vi "PDL_Process_AndSave.vi"(6 "Mergedata_struct":refnum<k24>[](array[refnum]), 7 "PDLSTS":refnum<k24>, 8 "错误输入（无错误）":errorcluster, 10 "PCU":refnum<k24>, 11 "chksavemu":bool) -> (0 "错误输出":errorcluster)   [LabVIEW 2017]
doc: "Save Measurement data"
uses:
  D:/test/PDLSTS/LV_PDL_Sample/DLL/STSProcess.dll
  DLL/STSProcess.dll
  D:/test/PDLSTS/LV_PDL_Sample/DLL/InstrumentDLL.dll
  DLL/InstrumentDLL.dll
panel:
  in  "SOPIL":dbl[][](array[numeric])
  in  "get_struct":refnum<k24>
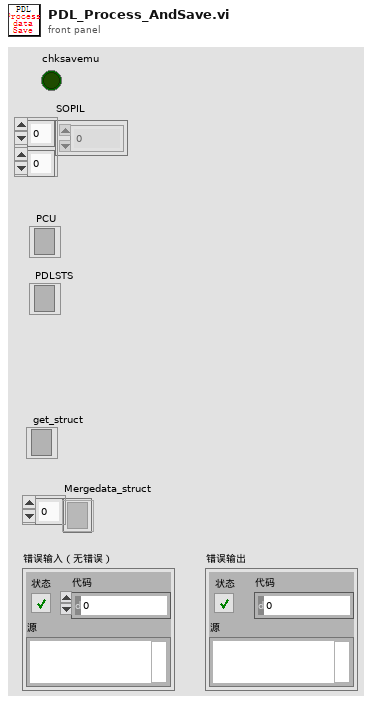
[diagram p1: front panel]
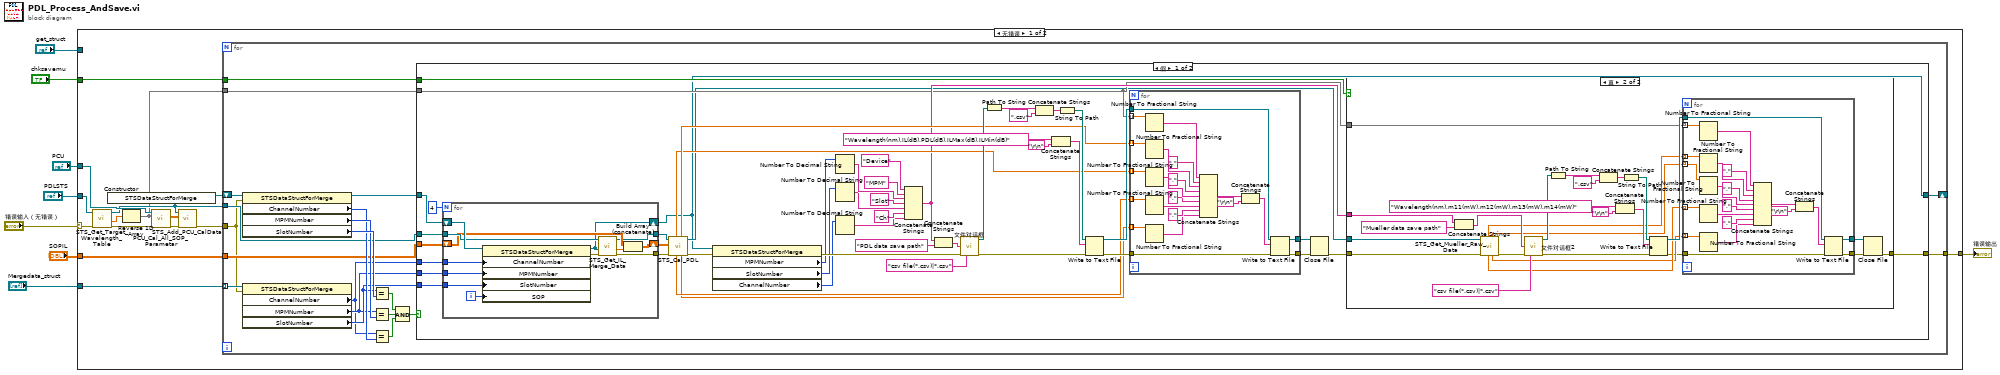
[diagram p0: block diagram]
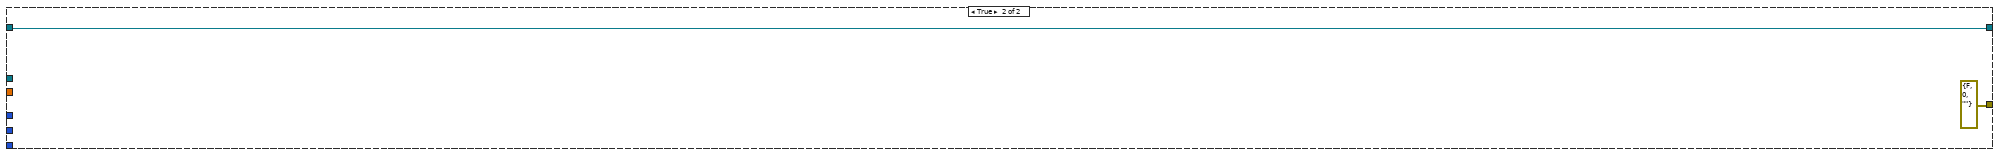
[diagram p3: hidden frame]
diagram:
  n1 = case shown="无错误" "错误输入（无错误）" {
    selector: "错误输入（无错误）" -> [w13 w177]
    tunnel: "Mergedata_struct" -> [w23 _]
    tunnel: "PDLSTS" -> [w22 _]
    tunnel: "PCU" -> [w20 _]
    tunnel: "get_struct" -> [_ _]
    tunnel: "SOPIL" -> [w16 _]
    tunnel: [w15 w177] -> w2
    tunnel: "chksavemu" -> [w12 _]
    frame No Error {
      n2 = call "STS_Get_Target_Wavelength_Table.vi"("错误输入（无错误）"=w13, ".NET引用句柄输入"=w22) -> ("error out"=w21:errorcluster, "wavelengths"=w10:dbl[], "引用输出"=w17:refnum<k24>)  [unwired: 7 in]
      n3 = constructor class="STSDataStructForMerge"() -> (reference out=w11:refnum<k24>)  [unwired: 3 in, 2 out]
      n4 = Reverse 1D Array(array=w10) -> (reversed array=w9:dbl[])
      n5 = call "PCU_Cal_All_SOP_Parametar.vi"("error in (no error)"=w21, "wave"=w9, ".NET Reference in"=w20) -> ("error out"=w19:errorcluster, "result out"=w18:sgl[][][])  [unwired: 6 in, 1 out]
      n6 = call "STS_Add_PCU_CalData.vi"("错误输入（无错误）"=w19, "errorArray"=w18, "STSProcess.PDLSTS"=w17) -> ("错误输出"=w14:errorcluster)  [unwired: 7 in, 1 out]
      n7 = for {
        tunnel: w17 -> [w31]
        tunnel: w23 -> [w43] mode=indexing
        tunnel: w16 -> [w30]
        tunnel: w9 -> [w29]
        tunnel: [w28] -> w15
        tunnel: w14 -> [w27]
        tunnel: w12 -> [w26]
        shift-right: [w25] -> _
        shift-left: w11 -> [w42]
        n8 = property class="STSDataStructForMerge"(reference=w42, error in=w27) -> (reference out=w24:refnum<k24>, "ChannelNumber"=w39:i32, "MPMNumber"=w40:i32, "SlotNumber"=w41:i32)  [unwired: 1 out]
        n9 = property class="STSDataStructForMerge"(reference=w43, error in=w27) -> ("ChannelNumber"=w32:i32, "MPMNumber"=w33:i32, "SlotNumber"=w34:i32)  [unwired: 2 out]
        n10 = Equal?(x=w34, y=w41) -> (x = y?=w38:bool)
        n11 = Equal?(x=w33, y=w40) -> (x = y?=w37:bool)
        n12 = Equal?(x=w32, y=w39) -> (x = y?=w36:bool)
        n13 = Compound Arithmetic op=AND ("复合运算")(w38, w37, w36) -> (w35:bool)
        n14 = case shown="假" w35 {
          tunnel: w24 -> [w91 w175]
          tunnel: w34 -> [w90 _]
          tunnel: w33 -> [w89 _]
          tunnel: w32 -> [w88 _]
          tunnel: w31 -> [w87 _]
          tunnel: w30 -> [w86 _]
          tunnel: w29 -> [w46 _]
          tunnel: [w48 errorcluster {"status"=FALSE, "code"=0, "source"=""} ("error out")] -> w28
          tunnel: w26 -> [w52 _]
          tunnel: [w44 w175] -> w25
          frame False {
            n15 = for {
              N: 4 -> [_]
              tunnel: w90 -> [w172]
              tunnel: w89 -> [w171]
              tunnel: w88 -> [w170]
              tunnel: w87 -> [w169]
              shift-right: [w165] -> w85
              shift-left: w86 -> [w166]
              tunnel: [w163] -> w84
              tunnel: [w162] -> w83
              shift-right: [w164] -> w44
              shift-left: w91 -> [w174]
              i -> [w173]
              n16 = property class="STSDataStructForMerge"(reference=w174, "ChannelNumber"=w170, "MPMNumber"=w171, "SlotNumber"=w172, "SOP"=w173) -> (reference out=w164:refnum<k24>, error out=w168:errorcluster)  [unwired: 1 in]
              n17 = call "STS_Get_IL_Merge_Data.vi"("错误输入（无错误）"=w168, "setting"=w164, ".NET引用句柄输入"=w169) -> ("error out"=w162:errorcluster, "ilData"=w167:sgl[], "引用输出"=w163:refnum<k24>)  [unwired: 6 in]
              n18 = Build Array (concatenate)(w166, w167) -> (w165:dbl[][])
            }
            n19 = call "STS_Cal_PDL.vi"("错误输入（无错误）"=w83, "ilData"=w85, ".NET引用句柄输入"=w84) -> ("error out"=w68:errorcluster, "引用输出"=w45:refnum<k24>, "minIL"=w53:sgl[], "il"=w56:sgl[], "maxIL"=w54:sgl[], "pdl"=w55:sgl[])  [unwired: 3 in]
            n20 = property on="属性节点" class="STSDataStructForMerge"(reference=w44, error in=w68) -> (error out=w75:errorcluster, "MPMNumber"=w65:i32, "SlotNumber"=w66:i32, "ChannelNumber"=w67:i32)  [unwired: 1 out]
            n21 = Number To Decimal String(number=w65) -> (decimal integer string=w63:string)  [unwired: 1 in]
            n22 = Number To Decimal String(number=w66) -> (decimal integer string=w61:string)  [unwired: 1 in]
            n23 = Number To Decimal String(number=w67) -> (decimal integer string=w59:string)  [unwired: 1 in]
            n24 = Concatenate Strings("Device", "MPM" ("字符串"), w63, "Slot" ("字符串"), w61, "Ch" ("字符串"), w59) -> (w47:string)
            n25 = Concatenate Strings(w47, "PDL data save path" ("字符串")) -> (w50:string)
            n26 = call "文件对话框"("default name"=w50, "error in"=w75, "pattern (all files)"="csv file(*.csv)|*.csv") -> ("selected path"=w79:path, "error out"=w74:errorcluster)  [unwired: 9 in, 2 out]
            n27 = Path To String(path=w79) -> (string=w78:string)
            n28 = Concatenate Strings(w78, ".csv" ("名称或相对路径")) -> (w77:string)
            n29 = Concatenate Strings("Wavelength(nm),IL(dB),PDL(dB),ILMax(dB),ILMin(dB)" ("字符串"), "\r\n") -> (w80:string)
            n30 = String To Path(string=w77) -> (path=w76:path)
            n31 = Write to Text File(file (use dialog)=w76, text=w80, error in=w74) -> (refnum out=w57:refnum<file>, error out=w58:errorcluster)  [unwired: 1 in, 1 out]
            n32 = for {
              tunnel: w46 -> [w161] mode=indexing
              tunnel: w58 -> [w159]
              tunnel: [w158] -> w81
              tunnel: w57 -> [w154]
              tunnel: [w153] -> w82
              tunnel: w56 -> [w148] mode=indexing
              tunnel: w55 -> [w147] mode=indexing
              tunnel: w54 -> [w145] mode=indexing
              tunnel: w53 -> [w141] mode=indexing
              n33 = Number To Fractional String(number=w161) -> (F-format string=w160:string)  [unwired: 3 in]
              n34 = Number To Fractional String(number=w148) -> (F-format string=w151:string)  [unwired: 3 in]
              n35 = Number To Fractional String(number=w147) -> (F-format string=w149:string)  [unwired: 3 in]
              n36 = Number To Fractional String(number=w145) -> (F-format string=w144:string)  [unwired: 3 in]
              n37 = Number To Fractional String(number=w141) -> (F-format string=w142:string)  [unwired: 3 in]
              n38 = Concatenate Strings(w160, "," ("字符串"), w151, "," ("字符串"), w149, "," ("字符串"), w144, "," ("字符串"), w142) -> (w157:string)
              n39 = Concatenate Strings(w157, "\r\n") -> (w155:string)
              n40 = Write to Text File(file (use dialog)=w154, text=w155, error in=w159) -> (refnum out=w153:refnum<file>, error out=w158:errorcluster)  [unwired: 1 in, 1 out]
            }
            n41 = Close File(refnum=w82, error in=w81) -> (error out=w49:errorcluster)  [unwired: 1 out]
            n42 = case shown="真" w52 {
              tunnel: w45 -> [_ w119]
              tunnel: w49 -> [w93 w118]
              tunnel: [w93 w94] -> w48
              tunnel: w47 -> [_ w115]
              tunnel: w46 -> [_ w102]
              frame False {
              }
              frame True {
                n43 = Concatenate Strings(w115, "Mueller data save path" ("字符串")) -> (w113:string)
                n44 = call "STS_Get_Mueller_Raw_Data.vi"("错误输入（无错误）"=w118, ".NET引用句柄输入"=w119) -> ("error out"=w112:errorcluster, "m14"=w98:dbl[], "m12"=w100:dbl[], "m13"=w99:dbl[], "m11"=w101:dbl[])  [unwired: 4 in, 1 out]
                n45 = call "文件对话框2"("default name"=w113, "error in"=w112, "pattern (all files)"="csv file(*.csv)|*.csv") -> ("selected path"=w108:path, "error out"=w117:errorcluster)  [unwired: 9 in, 2 out]
                n46 = Path To String(path=w108) -> (string=w111:string)
                n47 = Concatenate Strings(w111, ".csv" ("名称或相对路径")) -> (w110:string)
                n48 = Concatenate Strings("Wavelength(nm),m11(mW),m12(mW),m13(mW),m14(mW)" ("字符串"), "\r\n") -> (w104:string)
                n49 = String To Path(string=w110) -> (path=w107:path)
                n50 = Write to Text File(file (use dialog)=w107, text=w104, error in=w117) -> (refnum out=w103:refnum<file>, error out=w97:errorcluster)  [unwired: 1 in, 1 out]
                n51 = for {
                  tunnel: w102 -> [w140] mode=indexing
                  tunnel: w97 -> [w138]
                  tunnel: [w137] -> w96
                  tunnel: w103 -> [w133]
                  tunnel: [w132] -> w95
                  tunnel: w101 -> [w127] mode=indexing
                  tunnel: w100 -> [w126] mode=indexing
                  tunnel: w99 -> [w124] mode=indexing
                  tunnel: w98 -> [w120] mode=indexing
                  n52 = Number To Fractional String(number=w140) -> (F-format string=w139:string)  [unwired: 3 in]
                  n53 = Number To Fractional String(number=w127) -> (F-format string=w130:string)  [unwired: 3 in]
                  n54 = Number To Fractional String(number=w126) -> (F-format string=w128:string)  [unwired: 3 in]
                  n55 = Number To Fractional String(number=w124) -> (F-format string=w123:string)  [unwired: 3 in]
                  n56 = Number To Fractional String(number=w120) -> (F-format string=w121:string)  [unwired: 3 in]
                  n57 = Concatenate Strings(w139, "," ("字符串"), w130, "," ("字符串"), w128, "," ("字符串"), w123, "," ("字符串"), w121) -> (w136:string)
                  n58 = Concatenate Strings(w136, "\r\n") -> (w134:string)
                  n59 = Write to Text File(file (use dialog)=w133, text=w134, error in=w138) -> (refnum out=w132:refnum<file>, error out=w137:errorcluster)  [unwired: 1 in, 1 out]
                }
                n60 = Close File(refnum=w95, error in=w96) -> (error out=w94:errorcluster)  [unwired: 1 out]
              }
            }
          }
          frame True {
          }
        }
      }
    }
    frame Error {
    }
  }
  "错误输出" <- w2
